vi "Check Execution Result.vi"(8 "error in (no error)":errorcluster, 11 "Execution in":refnum<data-value>) -> (0 "error out":errorcluster, 2 "Execution Result":T1, 3 "Execution out":refnum<data-value>)   [LabVIEW 2015, in "Execution.lvclass"]
uses:
  Execution.lvclass
  EXECUTION_RESULT_TYPEDEF.ctl
  Step/STEP_STATUS.ctl
  Step.lvclass
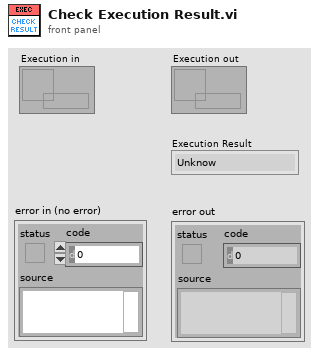
[diagram p1: front panel]
types:
  T1 = typedef "Execution.lvclass/EXECUTION_RESULT_TYPEDEF.ctl" = enum16{"Unknow", "Terminated", "Passed", "Failed", "Error"}
  T2 = typedef "Step.lvclass/STEP_STATUS.ctl" = enum16{"Skipped", "Done", "Passed", "Failed", "Error"}
  T3 = typedef "Execution.lvclass/STEP_RESULT.ctl" = cluster{"StepIndex":u32, "Step":refnum<class "Step.lvclass">, "StartTime":timestamp, "EndTime":timestamp, "Result":T2, "Error Info":string, "Measure Results":T4[]}
  T4 = typedef "Execution.lvclass/STEP_MEASURE_RESULT.ctl" = cluster{"Name":string, "Data Type":T5, "Check Type":T6, "String Limit":string, "Lower Limit":dbl, "Upper Limit":dbl, "Boolean Limit":bool, "Ignore Case":bool, "Measure Data":variant, "Result":T2, "Error Info":string}
  T5 = typedef "Step.lvclass/OUTPUT_DATA_TYPE.ctl" = enum16{"Boolean", "String", "Numeric", "Other"}
  T6 = typedef "Step.lvclass/OUTPUT_CHECK_TYPE.ctl" = enum16{"INVALID", "DO_NOT_CHECK", "RECORD", "VARIABLE", "EQUAL", "NOT_EQUAL", "STR_CONTAINS", "STR_START_WITH", "STR_END_WITH", "STR_REGEX_MATCH", "NUM_GT", "NUM_LT", "NUM_GE", "NUM_LE", "NUM_RANGE", "NUM_RANGE_BDY"}
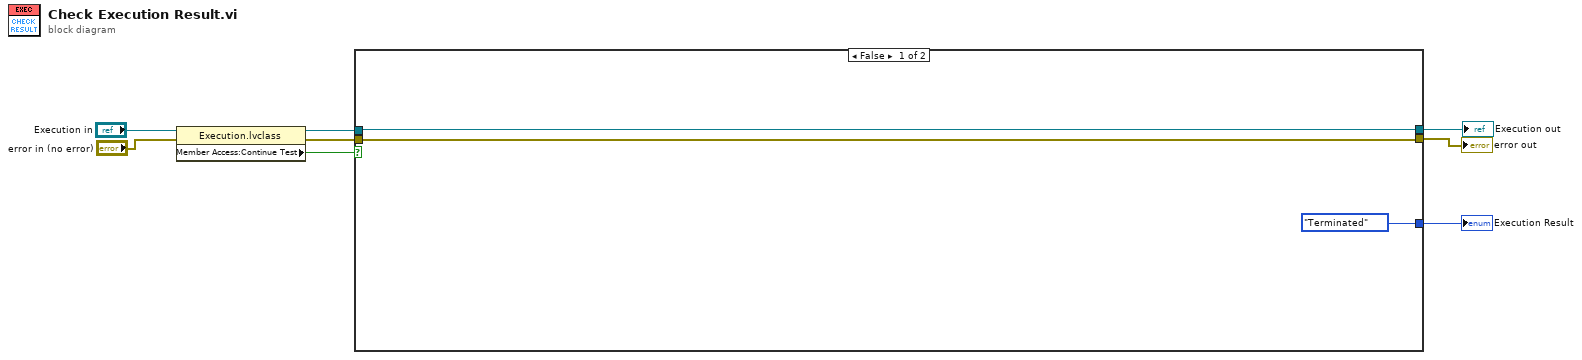
[diagram p0: block diagram]
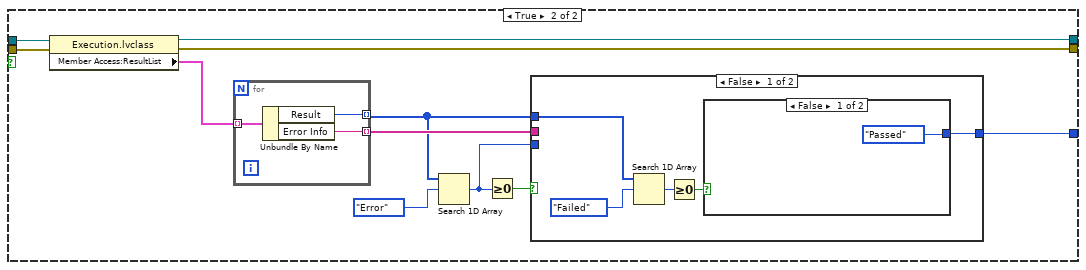
[diagram p2: hidden frame]
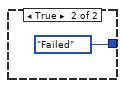
[diagram p3: hidden frame]
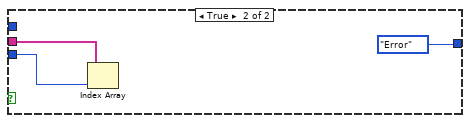
[diagram p4: hidden frame]
diagram:
  n1 = property class="Execution.lvclass"(reference="Execution in", error in="error in (no error)") -> (reference out=w6:refnum<data-value>, error out=w5:errorcluster, "Member Access:Continue Test"=w7:bool)
  n2 = case shown="False" w7 {
    tunnel: w6 -> [w10 w22]
    tunnel: w5 -> [w11 w21]
    tunnel: [EXECUTION_RESULT_TYPEDEF."Terminated" ("Execution Result") w14] -> w4
    tunnel: [w11 w13] -> w3
    tunnel: [w10 w12] -> w1
    frame False {
    }
    frame True {
      n3 = property class="Execution.lvclass"(reference=w22, error in=w21) -> (reference out=w12:refnum<data-value>, error out=w13:errorcluster, "Member Access:ResultList"=w20:T3[])
      n4 = for {
        tunnel: w20 -> [w35] mode=indexing
        tunnel: [w34] -> w15 mode=indexing
        tunnel: [w33] -> w17 mode=indexing
        n5 = Unbundle By Name(w35) -> ("Result"=w34:T2, "Error Info"=w33:string)
      }
      n6 = Search 1D Array(1D array=w15, element=STEP_STATUS."Error" ("Status")) -> (index of element=w16:i32)  [unwired: 1 in]
      n7 = Greater Or Equal To 0?(x=w16) -> (x >= 0?=w18:bool)
      n8 = case shown="False" w18 {
        tunnel: w17 -> [_ w32]
        tunnel: w16 -> [_ w31]
        tunnel: w15 -> [w26 _]
        tunnel: [w23 EXECUTION_RESULT_TYPEDEF."Error" ("Execution Result")] -> w14
        frame False {
          n9 = Search 1D Array(1D array=w26, element=STEP_STATUS."Failed" ("Status")) -> (index of element=w25:i32)  [unwired: 1 in]
          n10 = Greater Or Equal To 0?(x=w25) -> (x >= 0?=w24:bool)
          n11 = case shown="False" w24 {
            tunnel: [EXECUTION_RESULT_TYPEDEF."Passed" ("Execution Result") EXECUTION_RESULT_TYPEDEF."Failed" ("Execution Result")] -> w23
            frame False {
            }
            frame True {
            }
          }
        }
        frame True {
          n12 = Index Array(array=w32, index=w31) -> ()  [unwired: 1 out]
        }
      }
    }
  }
  "error out" <- w3
  "Execution Result" <- w4
  "Execution out" <- w1
